vi "RPC Method Register.vi"(8 "error in (no error)":errorcluster, 11 "OOP Server in":refnum<class "OOP Query Server.lvclass">) -> (0 "error out":errorcluster)   [LabVIEW 2019, in "OOP Query Server.lvlib" / "OOP Query Server.lvclass"]
uses:
  OOP Query Server.lvclass
  gRPC lvSupport/Server API/typeDefs/grpcId.ctl
  OOP Query Server.lvclass/OOP Query Server.ctl
  RPC Messages/ServerEvent/ServerEvent_Data.ctl
  gRPC lvSupport/gprc-lvsupport.lvlib
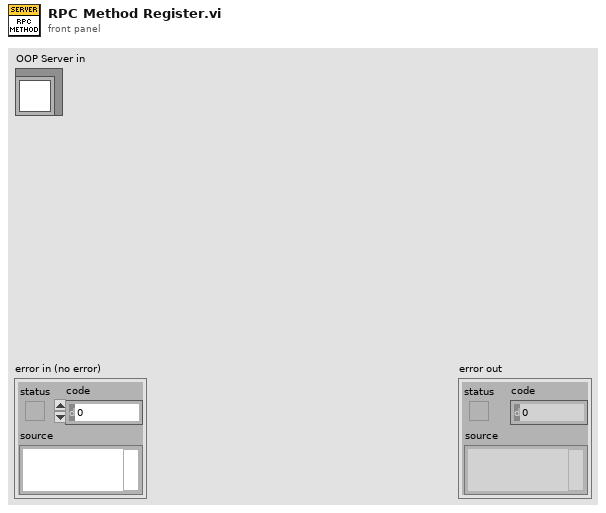
[diagram p1: front panel]
types:
  T1 = typedef "OOP Query Server.lvlib/gprc-lvsupport.lvlib/grpcId.ctl" = u64
  T2 = typedef "OOP Query Server.lvlib/OOP Query Server.lvclass/ServerEvent_Data.ctl" = cluster{"eventData":string, "serverId":i32, "status":i32}
  T3 = typedef "OOP Query Server.lvlib/OOP Query Server.lvclass/Server Internal UEs.ctl" = cluster{"Invoke Internal UE":refnum<user-event>, "Query Internal UE":refnum<user-event>, "Register Internal UE":refnum<user-event>}
  T4 = typedef "OOP Query Server.lvlib/OOP Query Server.lvclass/Server gRPC UEs.ctl" = cluster{"Invoke gRPC UE":refnum<user-event>, "Query gRPC UE":refnum<user-event>, "Register gRPC UE":refnum<user-event>}
  T5 = typedef "OOP Query Server.lvlib/OOP Query Server.lvclass/RegistrationRequest_Data.ctl" = cluster{"eventName":string}
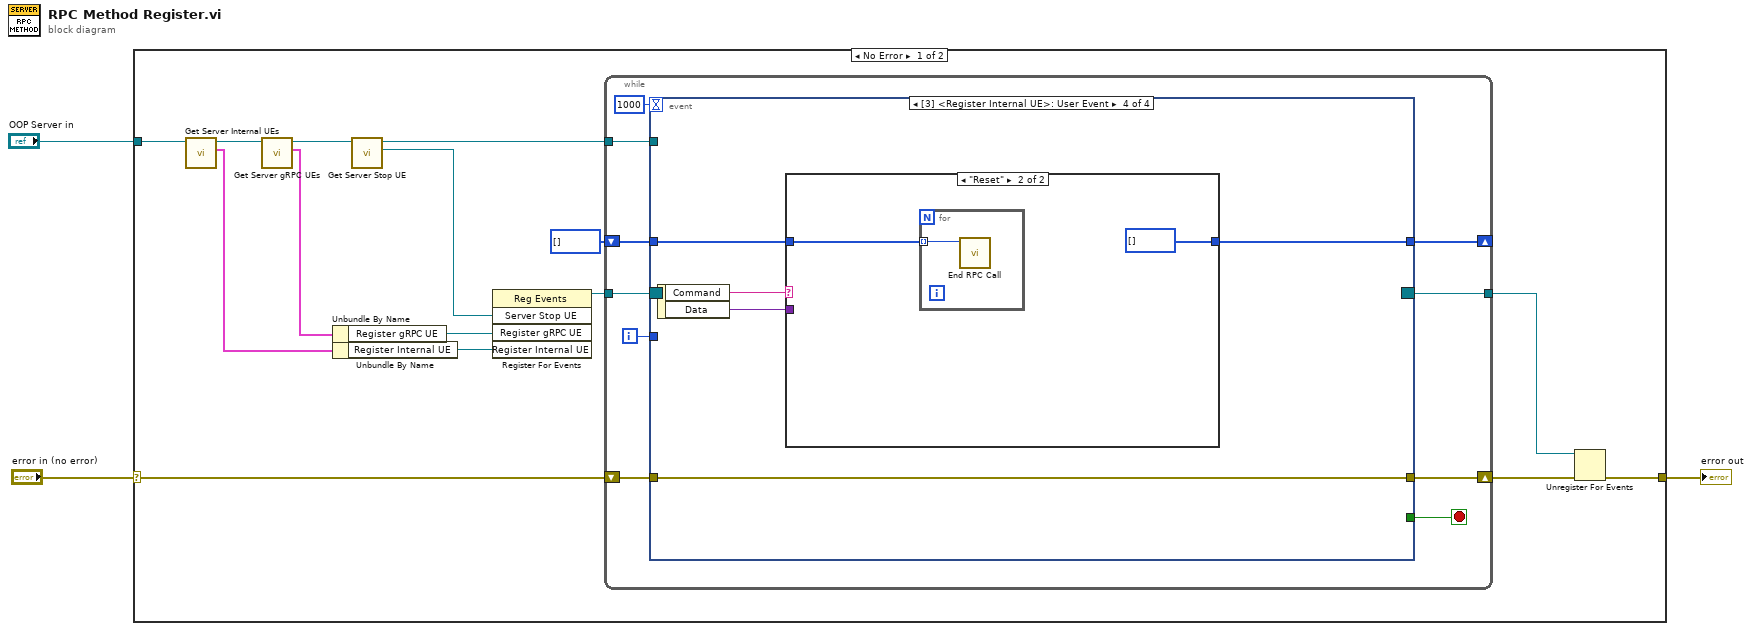
[diagram p0: block diagram]
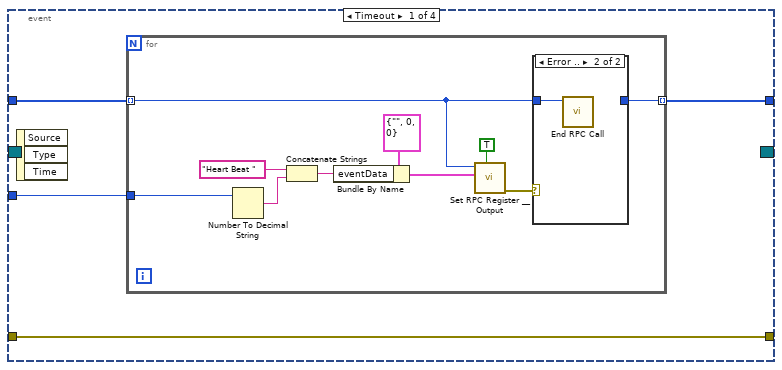
[diagram p2: hidden frame]
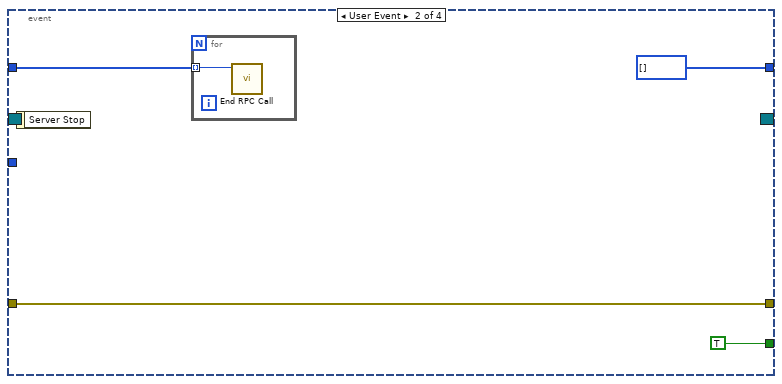
[diagram p4: hidden frame]
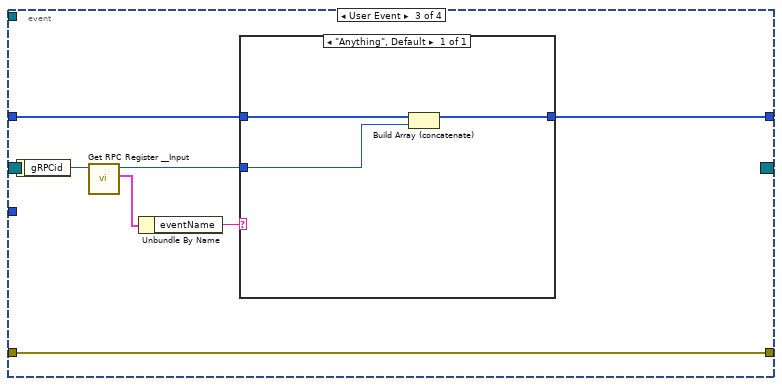
[diagram p5: hidden frame]
diagram:
  n1 = case shown="No Error" "error in (no error)" {
    selector: "error in (no error)" -> [w13 w69]
    tunnel: [w11 w69] -> w2
    tunnel: "OOP Server in" -> [w15 _]
    frame No Error {
      n2 = call "Get Server Internal UEs.vi"("OOP Server in"=w15) -> ("Server Internal UEs"=w7:T3, "OOP Server out"=w14:refnum<class "OOP Query Server.lvclass">)  [unwired: 9 in]
      n3 = call "Get Server gRPC UEs.vi"("OOP Server in"=w14) -> ("Server gRPC UEs"=w9:T4, "OOP Server out"=w18:refnum<class "OOP Query Server.lvclass">)  [unwired: 9 in]
      n4 = Unbundle By Name ("Unbundle gRPC UE")(w9) -> ("Register gRPC UE"=w8:refnum<user-event>)
      n5 = Unbundle By Name ("Unbundle Internal UE")(w7) -> ("Register Internal UE"=w6:refnum<user-event>)
      n6 = call "Get Server Stop UE.vi"("OOP Server in"=w18) -> ("Server Stop UE"=w17:refnum<user-event>, "OOP Server out"=w5:refnum<class "OOP Query Server.lvclass">)  [unwired: 9 in]
      n7 = register-events(w17, w8, w6) -> (reference out=w16:refnum<event-registration>)  [unwired: 2 in, 1 out]
      n8 = while {
        tunnel: w16 -> [w28]
        tunnel: [w24] -> w10
        shift-right: [w25] -> w12
        shift-left: w13 -> [w26]
        tunnel: w5 -> [w23]
        shift-right: [w20] -> _
        shift-left: T1[] [] -> [w22]
        i -> [w21]
        stop <- w27 stop-if-true
        n9 = event "RPC Method Event Structure" shown="[3] <Register Internal UE>: User Event" {
          selector: w28 -> [_ _ _ _]
          dyn-events: [_ _ _ _] -> w24
          timeout: 1000 -> [_ _ _ _]
          tunnel: [_ TRUE _ _] -> w27
          tunnel: w26 -> [w32 w47 w51 w60]
          tunnel: [w32 w47 w51 w60] -> w25
          tunnel: w23 -> [_ _ _ _]
          tunnel: w22 -> [w31 w46 w52 w62]
          tunnel: w21 -> [w30 _ _ _]
          tunnel: [w29 T1[] [] w50 w61] -> w20
          event Timeout {
            n10 = event-data() -> ()  [unwired: 1 in, 3 out]
            n11 = for {
              tunnel: w31 -> [w34] mode=indexing
              tunnel: w30 -> [w36]
              tunnel: [w33] -> w29 mode=indexing
              n12 = Number To Decimal String(number=w36) -> (decimal integer string=w40:string)  [unwired: 1 in]
              n13 = Concatenate Strings("Heart Beat " ("eventdata"), w40) -> (w38:string)
              n14 = Bundle By Name(cluster=T2 {"eventData"="", "serverId"=0, "status"=0} ("Message Data"), "eventData"=w38) -> (w37:T2)
              n15 = call "Set RPC Register __Output.vi"("Streeming? (F)"=TRUE, "Message Data"=w37, "gRPCid in"=w34) -> ("error out"=w35:errorcluster)  [unwired: 8 in]
              n16 = case shown="Error .." w35 {
                tunnel: w34 -> [w43 w44]
                tunnel: [w43 _] -> w33
                frame No Error {
                }
                frame Error {
                  n17 = call "End RPC Call.vi"("gRPCid"=w44) -> ()  [unwired: 10 in, 1 out]
                }
              }
            }
          }
          event User Event {
            n18 = event-data() -> ()  [unwired: 1 in, 1 out]
            n19 = for {
              tunnel: w46 -> [w49] mode=indexing
              n20 = call "End RPC Call.vi"("gRPCid"=w49) -> ()  [unwired: 10 in, 1 out]
            }
          }
          event User Event {
            n21 = event-data() -> ("gRPCid"=w56:T1)  [unwired: 1 in]
            n22 = call "Get RPC Register __Input.vi"("gRPCid in"=w56) -> ("Message Data"=w55:T5, "gRPCid out"=w53:T1)  [unwired: 8 in, 1 out]
            n23 = Unbundle By Name(w55) -> ("eventName"=w54:string)
            n24 = case shown="\"Anything\", Default" w54 {
              tunnel: w53 -> [w59]
              tunnel: [w58] -> w50
              tunnel: w52 -> [w57]
              frame "Anything", Default {
                n25 = Build Array (concatenate)(w57, w59) -> (w58:T1[])
              }
            }
          }
          event User Event {
            n26 = event-data() -> ("Command"=w64:string, "Data"=w63:variant)  [unwired: 1 in]
            n27 = case shown="\"Reset\"" w64 {
              tunnel: w63 -> [_ _]
              tunnel: w62 -> [w65 w67]
              tunnel: [w65 T1[] []] -> w61
              frame "None", Default {
              }
              frame "Reset" {
                n28 = for {
                  tunnel: w67 -> [w68] mode=indexing
                  n29 = call "End RPC Call.vi"("gRPCid"=w68) -> ()  [unwired: 10 in, 1 out]
                }
              }
            }
          }
        }
      }
      n30 = Unregister For Events(event registration refnum=w10, error in=w12) -> (error out=w11:errorcluster)
    }
    frame Error {
    }
  }
  "error out" <- w2
